vi "Type Color.vi"(11 "StringPanel in":refnum<class "StringPanel.lvclass">) -> (2 "Type Color":u32(colorbox))   [LabVIEW 2020, in "Conditum-Tools.lvlib" / "StringPanel.lvclass"]
uses:
  StringPanel.lvclass
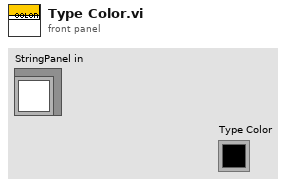
[diagram p1: front panel]
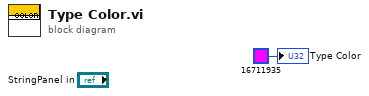
[diagram p0: block diagram]
diagram:
  "Type Color" <- u32 16711935 ("Type Color")
